vi "Port_get.vi"(8 "error in (no error)":errorcluster, 10 "Group":i32=1 min=1, 11 "OXY_SCPI Reseource In":refnum<visa-resource-name>) -> (0 "error out":errorcluster, 1 "communication_data":T1, 2 "Port":i32, 3 "OXY_SCPI Reseource Out":refnum<visa-resource-name>)   [LabVIEW 2020, in "OXYGEN_Datastream.lvlib"]
uses:
  OXYGEN_Datastream.lvlib
  TypeDefs/Cluster_RawCommData.ctl
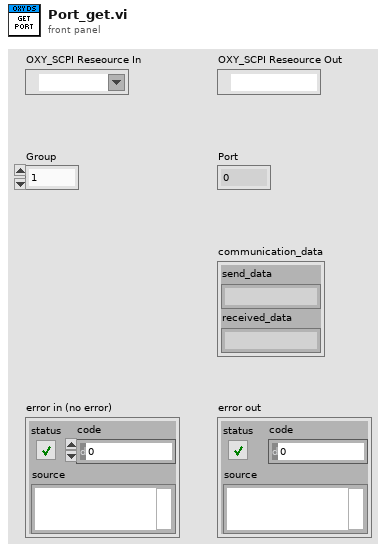
[diagram p1: front panel]
types:
  T1 = typedef "OXYGEN_Datastream.lvlib/Cluster_RawCommData.ctl" = cluster{"send_data":string, "received_data":string}
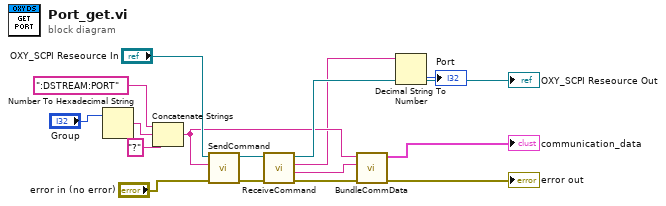
[diagram p0: block diagram]
diagram:
  n1 = Number To Hexadecimal String(2:"Group") -> (0:w7:string)  [unwired: 1 in]
  n2 = Concatenate Strings(":DSTREAM:PORT", w7, "?" ("string")) -> (w6:string)
  n3 = call "SendCommand.vi"("error in (no error)"="error in (no error)", "String to Send"=w6, "OXY_SCPI Reseource In"="OXY_SCPI Reseource In") -> ("error out"=w16:errorcluster, "OXY_SCPI Reseource Out"=w15:refnum<visa-resource-name>)  [unwired: 7 in]
  n4 = call "ReceiveCommand.vi"("error in (no error)"=w16, "OXY_SCPI Reseource In"=w15) -> ("error out"=w14:errorcluster, "received Data with Header"=w1:string, "received Data"=w3:string, "OXY_SCPI Reseource Out"=→"OXY_SCPI Reseource Out":refnum<visa-resource-name>)  [unwired: 6 in]
  n5 = call "BundleCommData.vi"("error in (no error)"=w14, "received_data"=w1, "send_data"=w6) -> ("error out"=→"error out":errorcluster, "communication_data"=→"communication_data":T1)  [unwired: 7 in]
  n6 = Decimal String To Number(string=w3) -> (number=→"Port":i32)  [unwired: 2 in, 1 out]
